vi "GetStepNamesFromPath.vi"(0 "path":string) -> (1 "Calib Step Name":string, 2 "Profile Step Name":string)   [LabVIEW 2009]
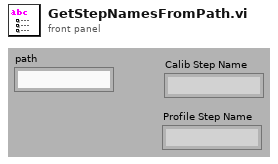
[diagram p1: front panel]
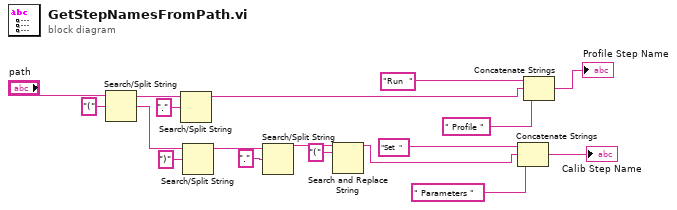
[diagram p0: block diagram]
diagram:
  n1 = Search/Split String(string="path", search string/char (-)="(") -> (substring before match=w3:string, match + rest of string=w5:string)  [unwired: 1 in, 1 out]
  n2 = Search/Split String(string=w3, search string/char (-)=".") -> (substring before match=w12:string)  [unwired: 1 in, 2 out]
  n3 = Search/Split String(string=w5, search string/char (-)=")") -> (substring before match=w8:string)  [unwired: 1 in, 2 out]
  n4 = Search/Split String(string=w8, search string/char (-)=".") -> (substring before match=w9:string)  [unwired: 1 in, 2 out]
  n5 = Search and Replace String(input string=w9, search string="(") -> (result string=w16:string)  [unwired: 6 in, 3 out]
  n6 = Concatenate Strings("Set  " ("search string/char (-)"), w16, " Parameters " ("search string/char (-)")) -> (→"Calib Step Name":string)
  n7 = Concatenate Strings("Run  " ("search string/char (-)"), w12, " Profile " ("search string/char (-)")) -> (→"Profile Step Name":string)
